vi "Car Wash.vi"() -> ()   [LabVIEW 2016, in "Car Wash.lvlib"]
uses:
  Car Wash.lvlib
  Controls/Car Wash Indicators.ctl
  Controls/Wash Options.ctl
  Controls/Queue Operations.ctl
  Controls/Data Cluster.ctl
  Controls/Timer Details.ctl
  Controls/Step Details.ctl
panel:
  out "Error Out":errorcluster
  in  "Start":bool
  out "Elapsed Time":dbl format="%0.2f"
  in  "stop":bool
  out "Wash Entry":bool
  in  "Wash Options":T1
  in  "Car Position":u8(slide) max=3 scale=0.0..4.0
  out "Car Wash Indicators":T2
  # "Entry Console"
  # "Car Wash Display"
  # "Car Position Simulation"
  # "Pre-Soak\nH-P Wash\nL-P Wax\nSpot Free Rinse"
  # "Underbody Wash\nBug Remover"
  # "Tire Shine\nAir Dry"
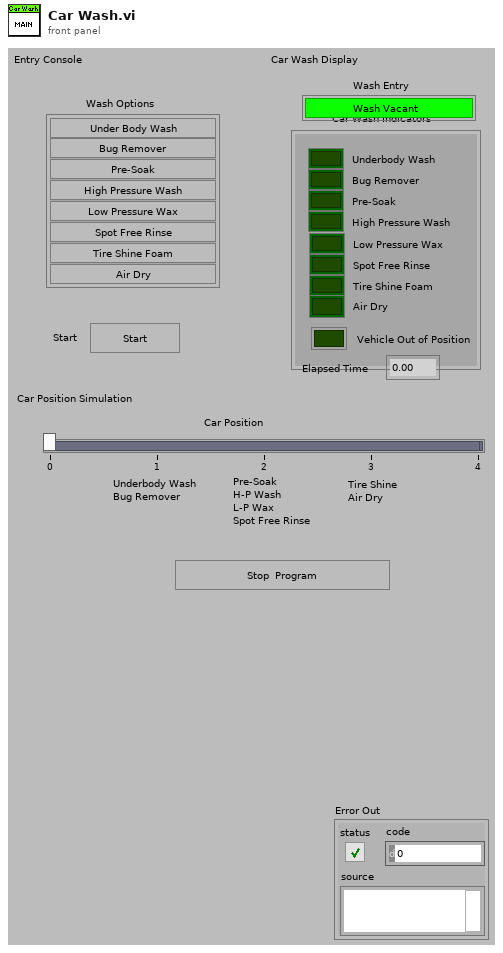
[diagram p1: front panel]
types:
  T1 = typedef "Car Wash.lvlib/Wash Options.ctl" = cluster{"Underbody Wash":bool, "Bug Remover":bool, "Pre-Soak":bool, "High Pressure Wash":bool, "Low Pressure Wax":bool, "Spot Free Rinse":bool, "Tire Shine Foam":bool, "Air Dry":bool}
  T2 = typedef "Car Wash.lvlib/Car Wash Indicators.ctl" = cluster{"Underbody Wash":bool, "Bug Remover":bool, "Pre-Soak":bool, "High Pressure Wash":bool, "Low Pressure Wax":bool, "Spot Free Rinse":bool, "Tire Shine Foam":bool, "Air Dry":bool, "Vehicle Out of Position":bool}
  T3 = typedef "Car Wash.lvlib/Data Cluster.ctl" = cluster{"Timer Details":T4, "Car Wash Indicators":T2, "Wash Options":T1, "Car Position Slider":u8, "Wash Entry":bool, "Enable Controls Ref":refnum<vi>[], "Disable Controls Ref":refnum<vi>[], "Steps Complete?":bool, "Selected Steps":T5[], "Current Step":T5, "Step Index (in selected)":i32, "Lookup":T5[]}
  T4 = typedef "Car Wash.lvlib/Timer Details.ctl" = cluster{"Paused?":bool, "Started?":bool, "Previous Time":timestamp, "Elapsed Time":dbl, "Set Time":dbl}
  T5 = typedef "Car Wash.lvlib/Step Details.ctl" = cluster{"Step":string, "Station":u8, "Time":dbl}
  T6 = typedef "Car Wash.lvlib/Queue Operations.ctl" = enum16{"Create", "Enqueue", "Enstack", "Dequeue", "Flush", "Release"}
  T7 = enum8{"Enabled", "Disabled", "Disabled and Grayed Out"}
  T8 = cluster{"Car Wash Indicators[0]":bool, "Car Wash Indicators[1]":bool, "Car Wash Indicators[2]":bool, "Car Wash Indicators[3]":bool, "Car Wash Indicators[4]":bool, "Car Wash Indicators[5]":bool, "Car Wash Indicators[6]":bool, "Car Wash Indicators[7]":bool, "Car Wash Indicators[8]":bool}
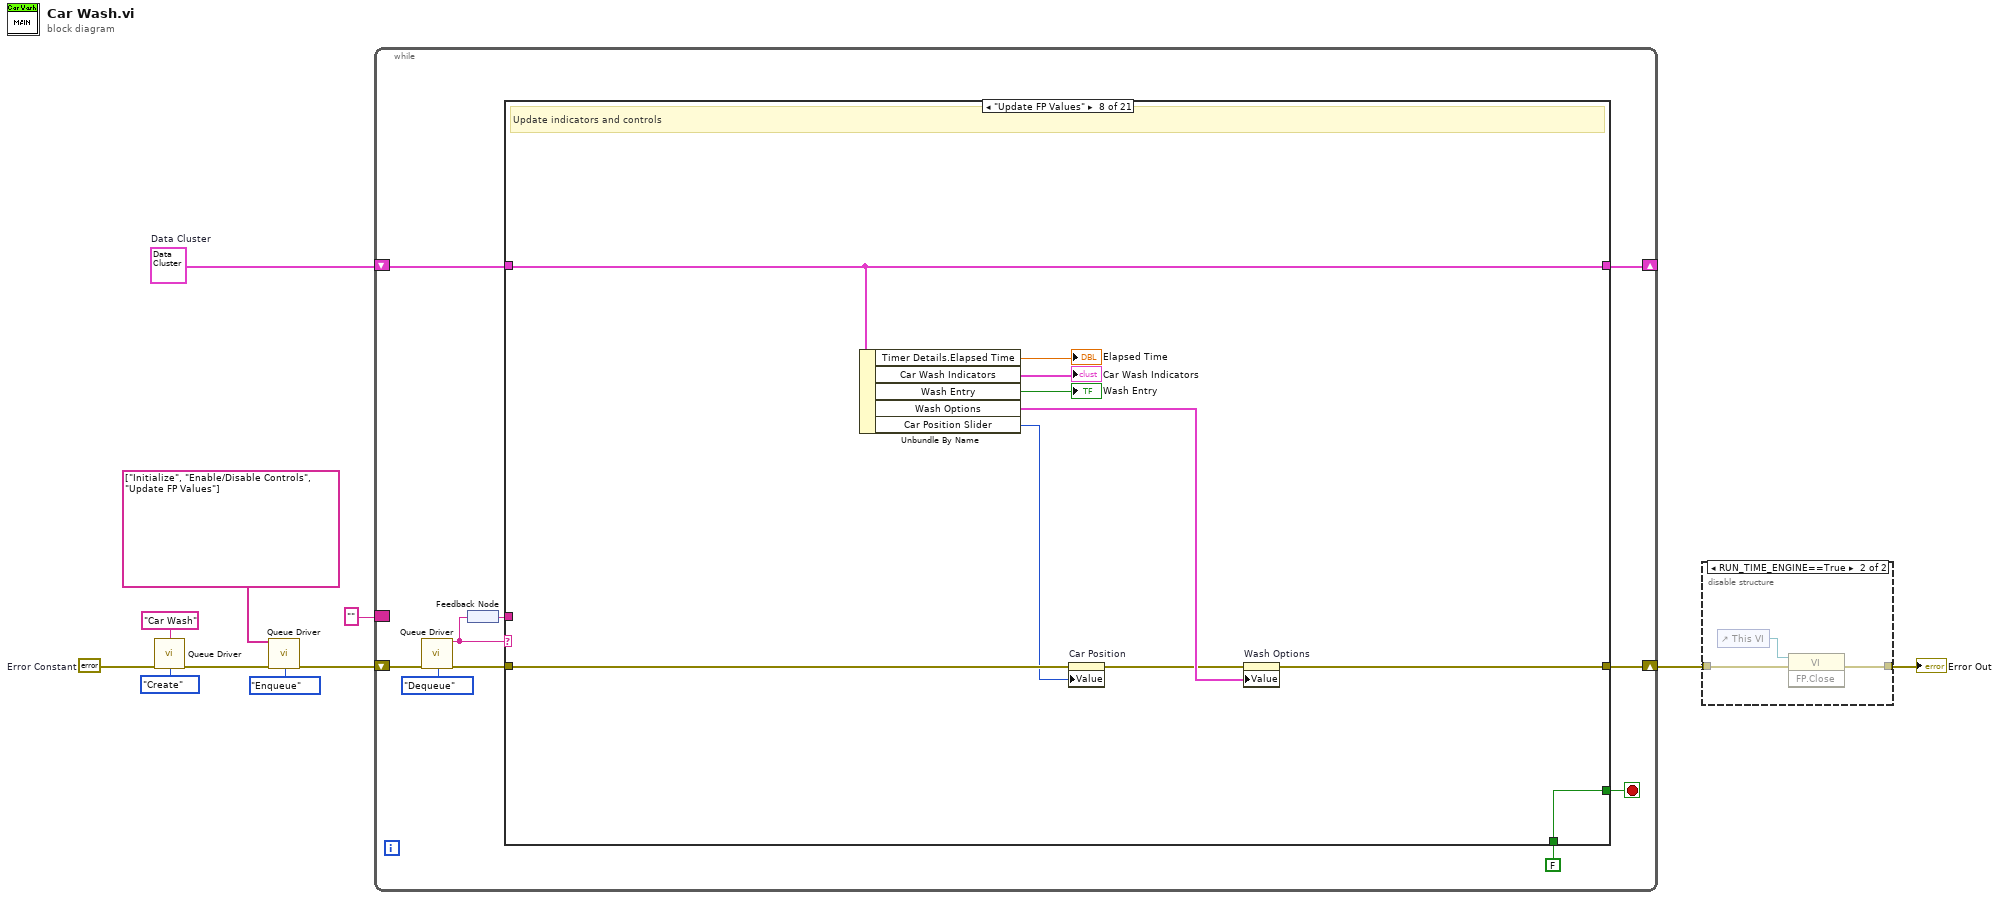
[diagram p0: block diagram]
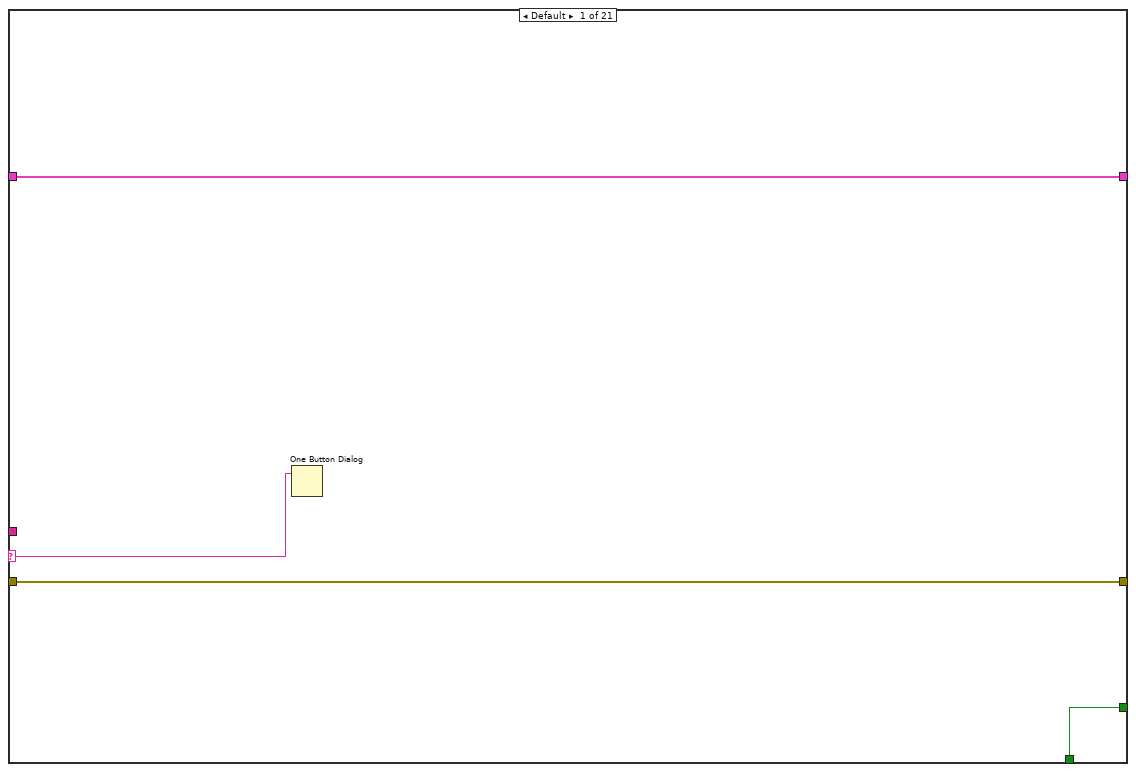
[diagram p2: hidden frame]
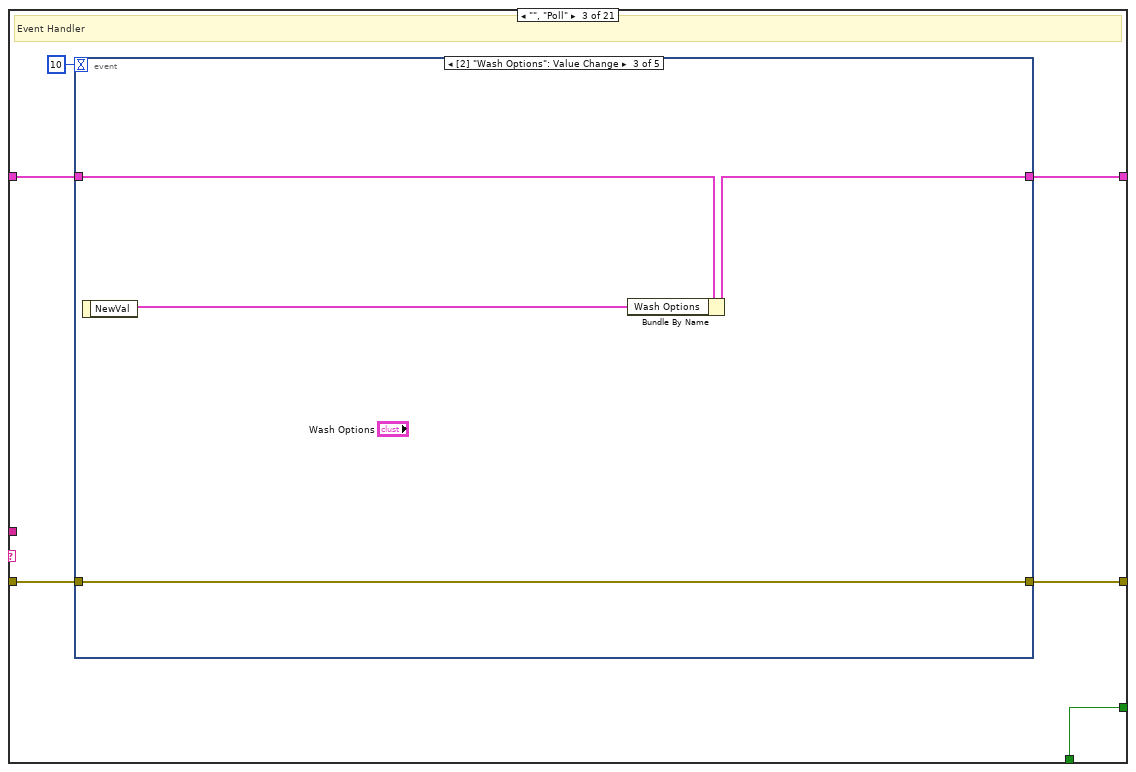
[diagram p4: hidden frame]
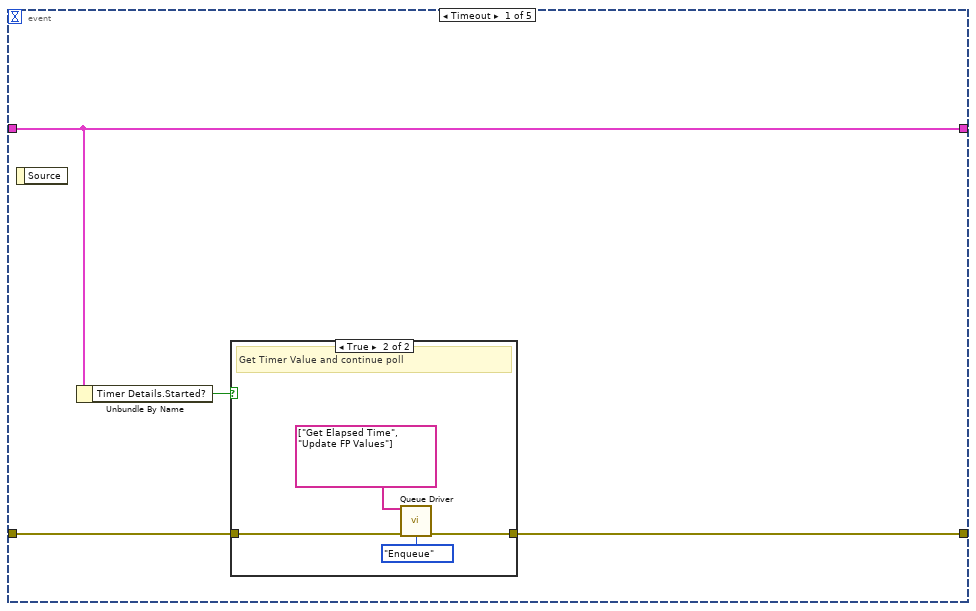
[diagram p5: hidden frame]
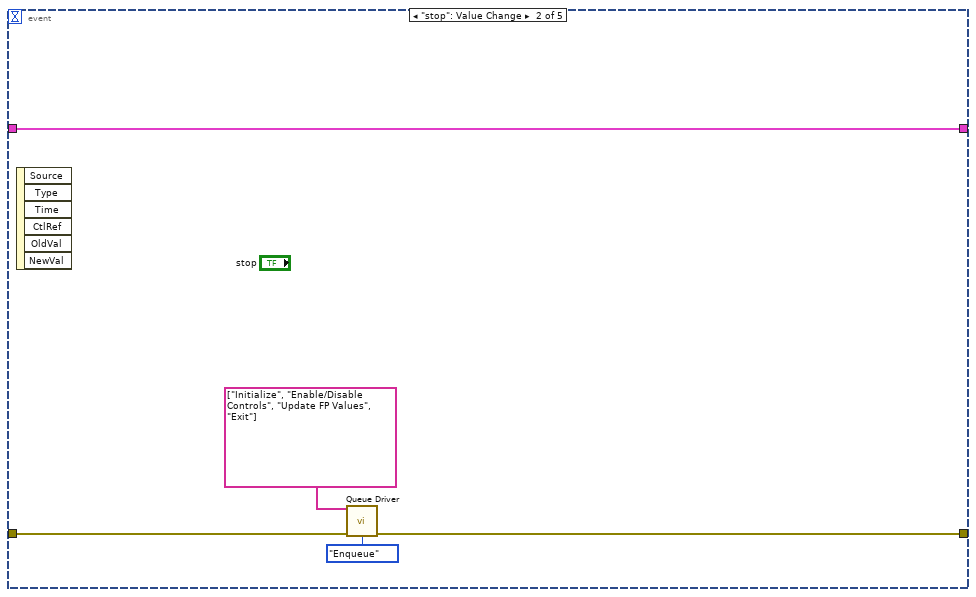
[diagram p7: hidden frame]
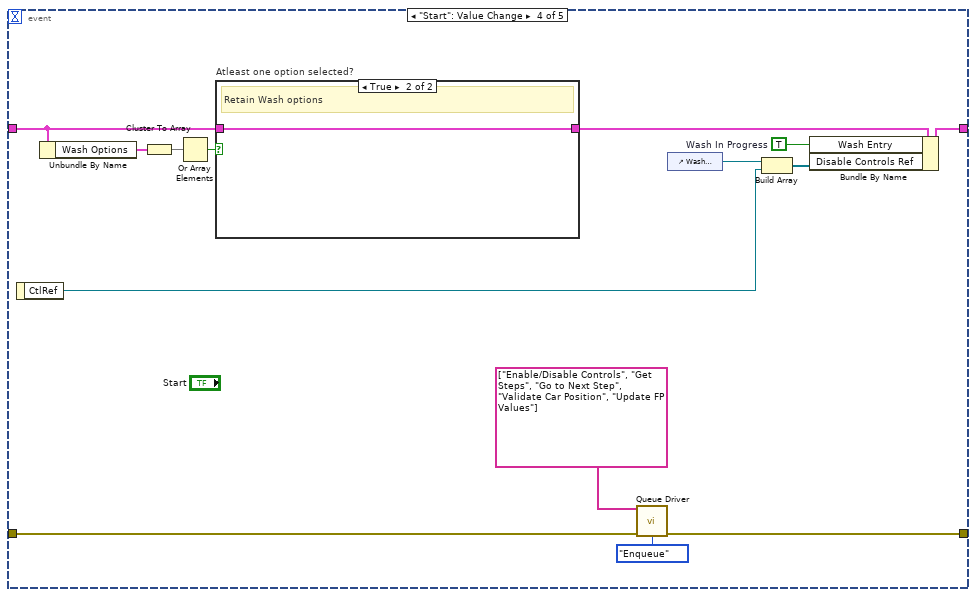
[diagram p8: hidden frame]
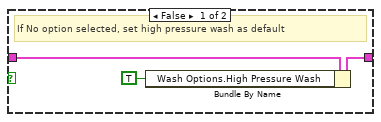
[diagram p9: hidden frame]
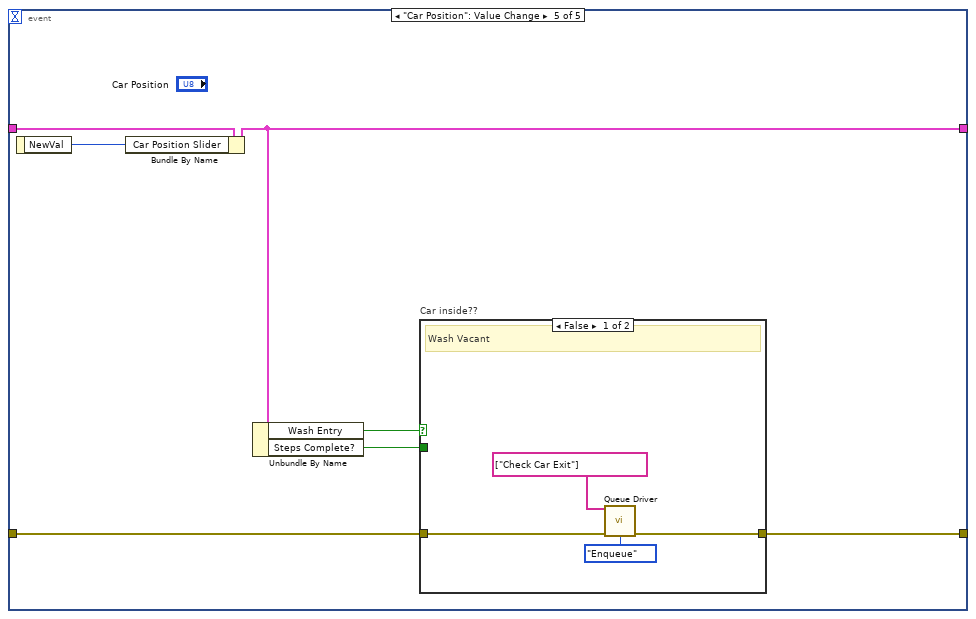
[diagram p10: hidden frame]
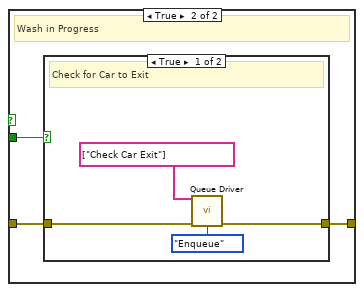
[diagram p11: hidden frame]
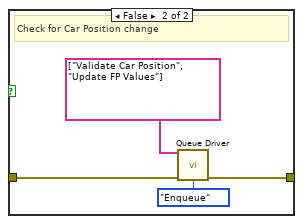
[diagram p12: hidden frame]
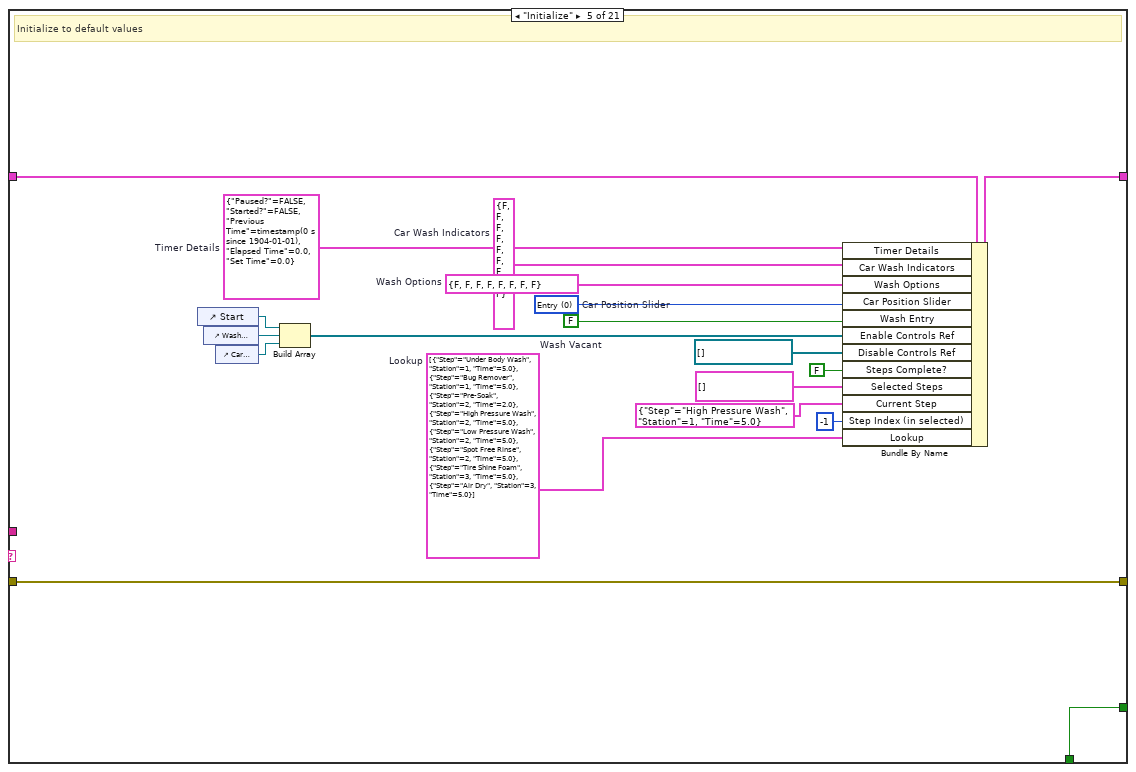
[diagram p14: hidden frame]
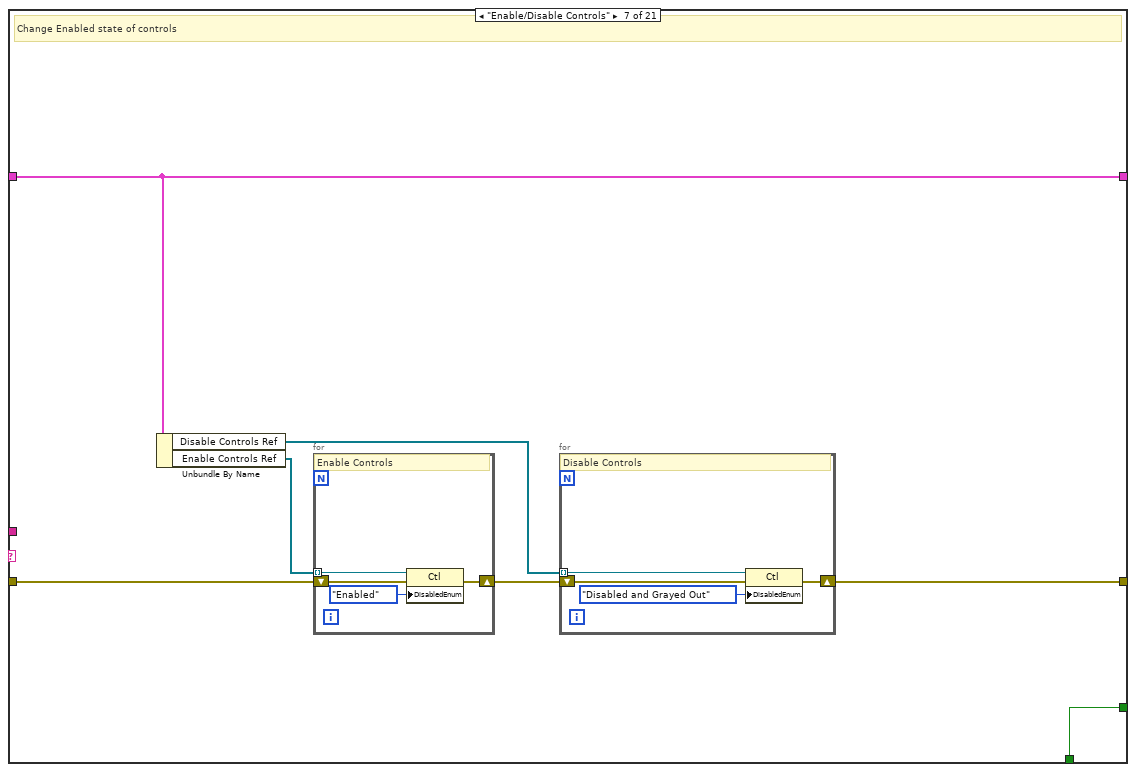
[diagram p16: hidden frame]
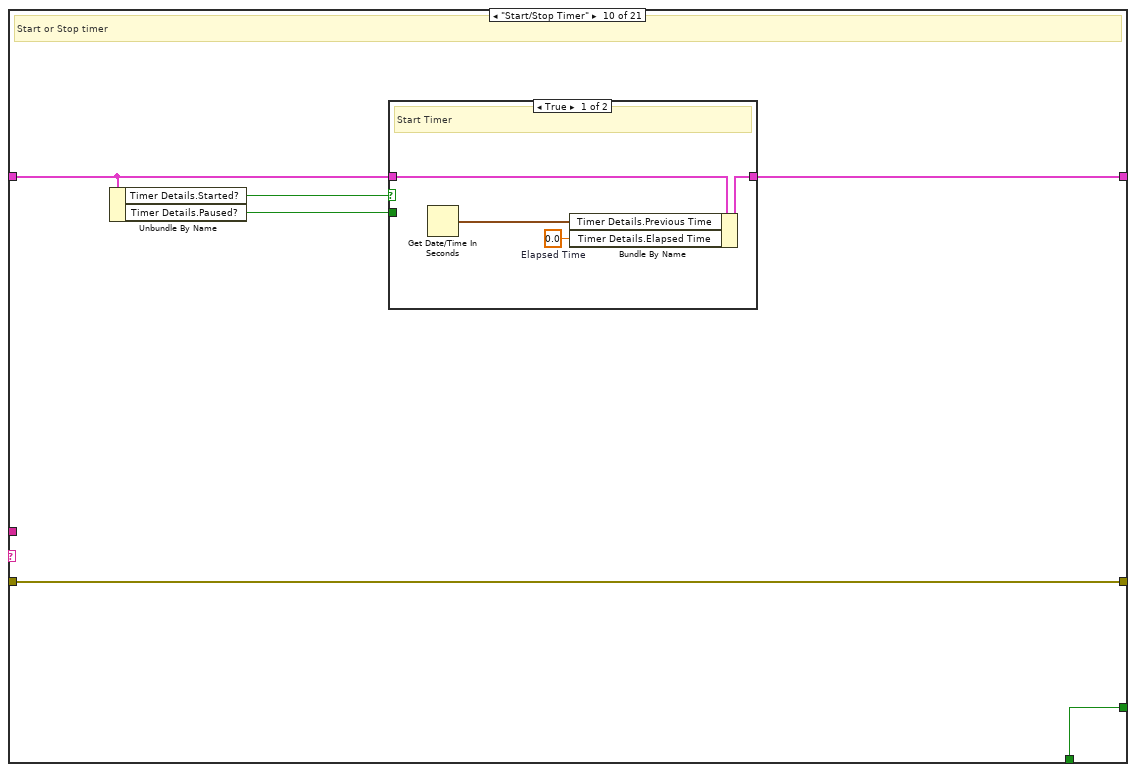
[diagram p18: hidden frame]
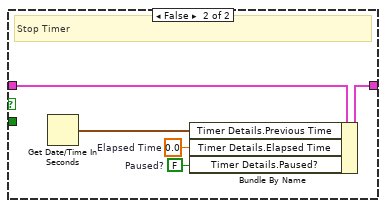
[diagram p19: hidden frame]
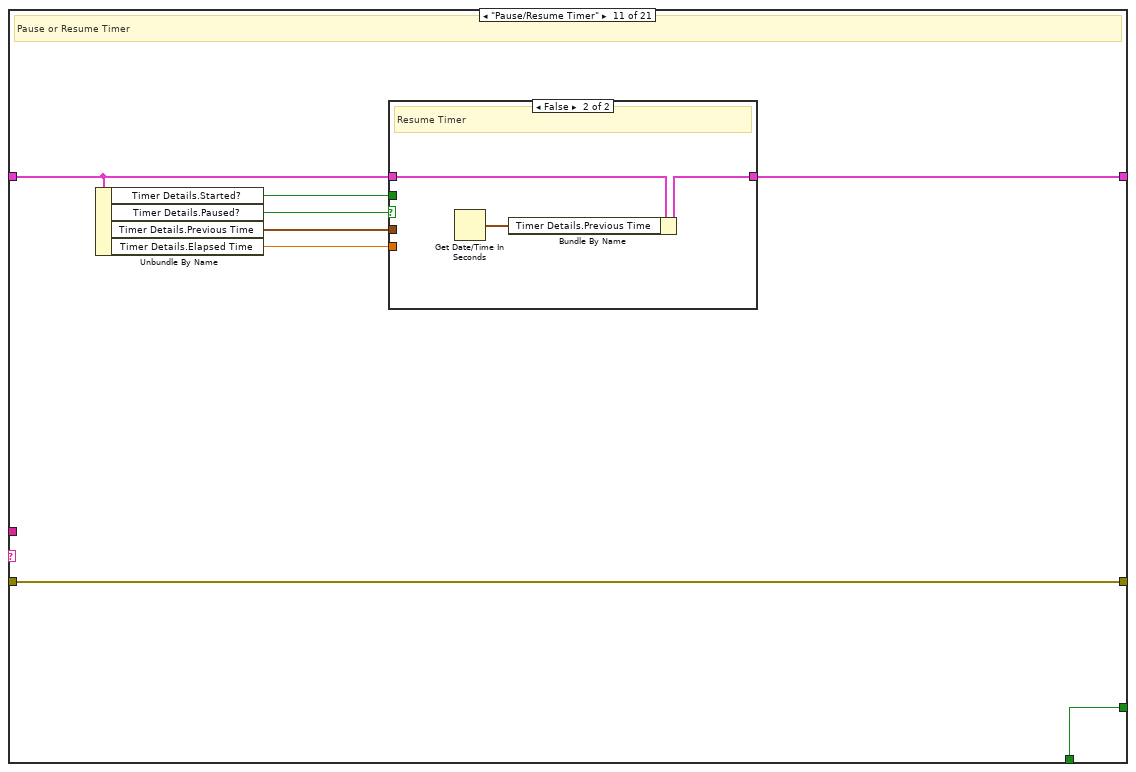
[diagram p20: hidden frame]
diagram:
  w3 = T3 {"Timer Details"={"Paused?"=FALSE, "Started?"=FALSE, "Previous Time"=timestamp(0 s since 1904-01-01), "Elapsed Time"=0.0, "Set Time"=0.0}, "Car Wash Indicators"={"Underbody Wash"=FALSE, "Bug Remover"=FALSE, "Pre-Soak"=FALSE, "High Pressure Wash"=FALSE, "Low Pressure Wax"=FALSE, "Spot Free Rinse"=FALSE, "Tire Shine Foam"=FALSE, "Air Dry"=FALSE, "Vehicle Out of Position"=FALSE}, "Wash Options"={"Underbody Wash"=FALSE, "Bug Remover"=FALSE, "Pre-Soak"=FALSE, "High Pressure Wash"=FALSE, "Low Pressure Wax"=FALSE, "Spot Free Rinse"=FALSE, "Tire Shine Foam"=FALSE, "Air Dry"=FALSE}, "Car Position Slider"=0, "Wash Entry"=FALSE, "Enable Controls Ref"=[], "Disable Controls Ref"=[], "Steps Complete?"=FALSE, "Selected Steps"=[], "Current Step"={"Step"="High Pressure Wash", "Station"=0, "Time"=0.0}, "Step Index (in selected)"=0, "Lookup"=[{"Step"="High Pressure Wash", "Station"=0, "Time"=0.0}, {"Step"="High Pressure Wash", "Station"=0, "Time"=0.0}, {"Step"="High Pressure Wash", "Station"=0, "Time"=0.0}, {"Step"="High Pressure Wash", "Station"=0, "Time"=0.0}, {"Step"="High Pressure Wash", "Station"=0, "Time"=0.0}, {"Step"="High Pressure Wash", "Station"=0, "Time"=0.0}, {"Step"="High Pressure Wash", "Station"=0, "Time"=0.0}, {"Step"="High Pressure Wash", "Station"=0, "Time"=0.0}]}  # Data Cluster
  w10 = errorcluster {"status"=FALSE, "code"=0, "source"=""}  # Error Constant
  n1 = call "Queue Driver.vi"("Queue Name"="Car Wash", "Error In"=w10, "Operation"=Queue_Operations."Create") -> ("Error Out"=w9:errorcluster)  [unwired: 11 in, 1 out]
  n2 = call "Queue Driver.vi"("Cases"=string[] ["Initialize", "Enable/Disable Controls", "Update FP Values"], "Error In"=w9, "Operation"=Queue_Operations."Enqueue") -> ("Error Out"=w8:errorcluster)  [unwired: 11 in, 1 out]
  n3 = while {
    shift-right: [w18] -> w2
    shift-left: w8 -> [w17]
    border: "" ("Dequeued Case") -> [_]
    shift-right: [w13] -> _
    shift-left: w3 -> [w14]
    stop <- w21 stop-if-true
    n4 = call "Queue Driver.vi"("Error In"=w17, "Operation"=Queue_Operations."Dequeue") -> ("Dequeued Case"=w16:string, "Error Out"=w19:errorcluster)  [unwired: 12 in]
    n5 = feedback #1() -> (w15:string)
    n6 = feedback-in #1(w16) -> ()
    n7 = case shown="\"Update FP Values\"" w16 {
      selector: w16 -> [w22 _ _ _ _ _ _ _ _ _ _ _ _ _ _ _ _ _ _ _ _]
      tunnel: FALSE -> [w25 w28 w34 w95 w114 w117 w124 w142 w145 w151 w168 w188 w203 w212 w226 w273 w301 w309 w323 w333 _]
      tunnel: [w25 w28 w34 w95 w114 w117 w124 w142 w145 w151 w168 w188 w203 w212 w226 w273 w301 w309 w323 w333 TRUE] -> w21
      tunnel: w19 -> [w24 w27 w33 w94 w113 w116 w121 w141 w144 w150 w167 w179 w202 w211 w220 w270 w298 w308 w322 w332 w340]
      tunnel: [w24 w27 w32 w94 w113 w116 w119 w136 w144 w150 w167 w178 w202 w211 w219 w269 w297 w308 w321 w332 w338] -> w18
      tunnel: w15 -> [_ _ _ _ _ _ _ _ _ _ _ _ _ _ _ _ _ _ w310 _ _]
      tunnel: w14 -> [w23 w26 w31 w93 w112 w115 w123 w140 w143 w147 w166 w185 w201 w207 w222 w272 w300 w307 w311 w331 w334]
      tunnel: [w23 w26 w30 w93 w111 w115 w123 w140 w143 w146 w165 w184 w201 w206 w221 w271 w300 w307 w311 w331 w334] -> w13
      frame Default {
        n8 = One Button Dialog(message=w22) -> ()  [unwired: 1 in, 1 out]
      }
      frame "----Poll----" {
      }
      frame "", "Poll" {
        # "Event Handler"
        n9 = event shown="[2] \"Wash Options\": Value Change" {
          selector: _ -> [_ _ _ _ _]
          dyn-events: _ -> [_ _ _ _ _]
          timeout: 10 -> [_ _ _ _ _]
          tunnel: w33 -> [w38 w47 w49 w60 w75]
          tunnel: [w37 w46 w49 w59 w74] -> w32
          tunnel: w31 -> [w36 w44 w52 w65 w77]
          tunnel: [w36 w44 w51 w57 w73] -> w30
          event Timeout {
            n10 = event-data() -> ()  [unwired: 1 in, 1 out]
            n11 = Unbundle By Name(w36) -> ("Timer Details.Started?"=w35:bool)
            n12 = case shown="True" w35 {
              tunnel: w38 -> [w39 w43]
              tunnel: [w39 w42] -> w37
              frame False {
                # "Timer Not Running, so keep polling"
              }
              frame True {
                # "Get Timer Value and continue poll"
                n13 = call "Queue Driver.vi"("Cases"=string[] ["Get Elapsed Time", "Update FP Values"], "Error In"=w43, "Operation"=Queue_Operations."Enqueue") -> ("Error Out"=w42:errorcluster)  [unwired: 11 in, 1 out]
              }
            }
          }
          event "stop": Value Change {
            n14 = event-data() -> ()  [unwired: 1 in, 6 out]
            n15 = call "Queue Driver.vi"("Cases"=string[] ["Initialize", "Enable/Disable Controls", "Update FP Values", "Exit"], "Error In"=w47, "Operation"=Queue_Operations."Enqueue") -> ("Error Out"=w46:errorcluster)  [unwired: 11 in, 1 out]
          }
          event Value Change {
            n16 = event-data() -> ("NewVal"=w50:T1)  [unwired: 1 in]
            n17 = Bundle By Name(cluster=w52, "Wash Options"=w50) -> (w51:T3)
          }
          event "Start": Value Change {
            w56 = TRUE  # Wash In Progress
            n18 = event-data() -> ("CtlRef"=w53:refnum<vi>)  [unwired: 1 in]
            n19 = Unbundle By Name(w65) -> ("Wash Options"=w63:T1)
            n20 = Cluster To Array(cluster=w63) -> (array=w64:bool[])
            n21 = Or Array Elements(Boolean array=w64) -> (logical OR=w62:bool)
            n22 = case "Atleast one option selected?" shown="True" w62 {
              tunnel: [w69 w70] -> w66
              tunnel: w65 -> [w68 w70]
              frame False {
                # "If No option selected, set high pressure wash as default"
                n23 = Bundle By Name(cluster=w68, "Wash Options.High Pressure Wash"=TRUE) -> (w69:T3)
              }
              frame True {
                # "Retain Wash options"
              }
            }
            n24 = call "Queue Driver.vi"("Cases"=string[] ["Enable/Disable Controls", "Get Steps", "Go to Next Step", "Validate Car Position", "Update FP Values"], "Error In"=w60, "Operation"=Queue_Operations."Enqueue") -> ("Error Out"=w59:errorcluster)  [unwired: 11 in, 1 out]
            n25 = control-ref of="Wash Options"() -> (w55:refnum<vi>)
            n26 = Build Array(w55, w53) -> (w54:refnum<vi>[])
            n27 = Bundle By Name(cluster=w66, "Wash Entry"=w56, "Disable Controls Ref"=w54) -> (w57:T3)
          }
          event "Car Position": Value Change {
            n28 = event-data() -> ("NewVal"=w76:u8)  [unwired: 1 in]
            n29 = Bundle By Name(cluster=w77, "Car Position Slider"=w76) -> (w73:T3)
            n30 = Unbundle By Name(w73) -> ("Wash Entry"=w71:bool, "Steps Complete?"=w72:bool)
            n31 = case "Car inside??" shown="False" w71 {
              tunnel: w75 -> [w81 w84]
              tunnel: [w80 w83] -> w74
              tunnel: w72 -> [_ w82]
              frame False {
                # "Wash Vacant"
                n32 = call "Queue Driver.vi"("Cases"=string[] ["Check Car Exit"], "Error In"=w81, "Operation"=Queue_Operations."Enqueue") -> ("Error Out"=w80:errorcluster)  [unwired: 11 in, 1 out]
              }
              frame True {
                # "Wash in Progress"
                n33 = case shown="True" w82 {
                  tunnel: w84 -> [w86 w90]
                  tunnel: [w85 w89] -> w83
                  frame True {
                    # "Check for Car to Exit"
                    n34 = call "Queue Driver.vi"("Cases"=string[] ["Check Car Exit"], "Error In"=w86, "Operation"=Queue_Operations."Enqueue") -> ("Error Out"=w85:errorcluster)  [unwired: 11 in, 1 out]
                  }
                  frame False {
                    # "Check for Car Position change"
                    n35 = call "Queue Driver.vi"("Cases"=string[] ["Validate Car Position", "Update FP Values"], "Error In"=w90, "Operation"=Queue_Operations."Enqueue") -> ("Error Out"=w89:errorcluster)  [unwired: 11 in, 1 out]
                  }
                }
              }
            }
          }
        }
      }
      frame "----Initialize----" {
      }
      frame "Initialize" {
        w96 = T5[] [{"Step"="Under Body Wash", "Station"=1, "Time"=5.0}, {"Step"="Bug Remover", "Station"=1, "Time"=5.0}, {"Step"="Pre-Soak", "Station"=2, "Time"=2.0}, {"Step"="High Pressure Wash", "Station"=2, "Time"=5.0}, {"Step"="Low Pressure Wash", "Station"=2, "Time"=5.0}, {"Step"="Spot Free Rinse", "Station"=2, "Time"=5.0}, {"Step"="Tire Shine Foam", "Station"=3, "Time"=5.0}, {"Step"="Air Dry", "Station"=3, "Time"=5.0}]  # Lookup
        w106 = FALSE  # Wash Vacant
        w107 = u8 0 items=["Entry", "Station 1", "Station 2", "Station 3", "Exit"]  # Car Position Slider
        w108 = T1 {"Underbody Wash"=FALSE, "Bug Remover"=FALSE, "Pre-Soak"=FALSE, "High Pressure Wash"=FALSE, "Low Pressure Wax"=FALSE, "Spot Free Rinse"=FALSE, "Tire Shine Foam"=FALSE, "Air Dry"=FALSE}  # Wash Options
        w109 = T2 {"Underbody Wash"=FALSE, "Bug Remover"=FALSE, "Pre-Soak"=FALSE, "High Pressure Wash"=FALSE, "Low Pressure Wax"=FALSE, "Spot Free Rinse"=FALSE, "Tire Shine Foam"=FALSE, "Air Dry"=FALSE, "Vehicle Out of Position"=FALSE}  # Car Wash Indicators
        w110 = T4 {"Paused?"=FALSE, "Started?"=FALSE, "Previous Time"=timestamp(0 s since 1904-01-01), "Elapsed Time"=0.0, "Set Time"=0.0}  # Timer Details
        # "Initialize to default values"
        n36 = control-ref of="Start"() -> (w103:refnum<vi>)
        n37 = control-ref of="Wash Options"() -> (w105:refnum<vi>)
        n38 = control-ref of="Car Position"() -> (w104:refnum<vi>)
        n39 = Build Array(w103, w105, w104) -> (w102:refnum<vi>[])
        n40 = Bundle By Name(cluster=w112, "Timer Details"=w110, "Car Wash Indicators"=w109, "Wash Options"=w108, "Car Position Slider"=w107, "Wash Entry"=w106, "Enable Controls Ref"=w102, "Disable Controls Ref"=refnum<vi>[] [], "Steps Complete?"=FALSE, "Selected Steps"=T5[] [], "Current Step"=T5 {"Step"="High Pressure Wash", "Station"=1, "Time"=5.0}, "Step Index (in selected)"=-1, "Lookup"=w96) -> (w111:T3)
      }
      frame "----FP Related----" {
      }
      frame "Enable/Disable Controls" {
        # "Change Enabled state of controls"
        n41 = Unbundle By Name(w123) -> ("Disable Controls Ref"=w118:refnum<vi>[], "Enable Controls Ref"=w122:refnum<vi>[])
        n42 = for {
          tunnel: w122 -> [w132] mode=indexing
          shift-right: [w129] -> w120
          shift-left: w121 -> [w131]
          # "Enable Controls"
          n43 = property class="Ctl"(reference=w132, error in=w131, "DisabledEnum"=T7."Enabled" ("Disabled")) -> (error out=w129:errorcluster)  [unwired: 1 out]
        }
        n44 = for {
          tunnel: w118 -> [w128] mode=indexing
          shift-right: [w125] -> w119
          shift-left: w120 -> [w127]
          # "Disable Controls"
          n45 = property class="Ctl"(reference=w128, error in=w127, "DisabledEnum"=T7."Disabled and Grayed Out" ("Disabled")) -> (error out=w125:errorcluster)  [unwired: 1 out]
        }
      }
      frame "Update FP Values" {
        # "Update indicators and controls"
        n46 = Unbundle By Name(w140) -> ("Timer Details.Elapsed Time"=→"Elapsed Time":dbl, "Car Wash Indicators"=→"Car Wash Indicators":T2, "Wash Entry"=→"Wash Entry":bool, "Wash Options"=w135:T1, "Car Position Slider"=w133:u8)
        n47 = property on="Car Position" class="Slide (strict)"(error in=w141, "Value"=w133) -> (error out=w134:errorcluster)  [unwired: 1 in, 1 out]
        n48 = property on="Wash Options" class="Clust (strict)"(error in=w134, "Value"=w135) -> (error out=w136:errorcluster)  [unwired: 1 in, 1 out]
      }
      frame "----Timer----" {
      }
      frame "Start/Stop Timer" {
        # "Start or Stop timer"
        n49 = Unbundle By Name(w147) -> ("Timer Details.Started?"=w149:bool, "Timer Details.Paused?"=w148:bool)
        n50 = case shown="True" w149 {
          tunnel: w148 -> [_ _]
          tunnel: w147 -> [w155 w160]
          tunnel: [w154 w159] -> w146
          frame True {
            w152 = 0.0  # Elapsed Time
            # "Start Timer"
            n51 = Get Date/Time In Seconds() -> (seconds since 1Jan1904=w153:timestamp)
            n52 = Bundle By Name(cluster=w155, "Timer Details.Previous Time"=w153, "Timer Details.Elapsed Time"=w152) -> (w154:T3)
          }
          frame False {
            w156 = FALSE  # Paused?
            w157 = 0.0  # Elapsed Time
            # "Stop Timer"
            n53 = Get Date/Time In Seconds() -> (seconds since 1Jan1904=w158:timestamp)
            n54 = Bundle By Name(cluster=w160, "Timer Details.Previous Time"=w158, "Timer Details.Elapsed Time"=w157, "Timer Details.Paused?"=w156) -> (w159:T3)
          }
        }
      }
      frame "Pause/Resume Timer" {
        # "Pause or Resume Timer"
        n55 = Unbundle By Name(w166) -> ("Timer Details.Started?"=w162:bool, "Timer Details.Paused?"=w161:bool, "Timer Details.Previous Time"=w164:timestamp, "Timer Details.Elapsed Time"=w163:dbl)
        n56 = case shown="False" w161 {
          tunnel: w166 -> [w172 w175]
          tunnel: [w171 w174] -> w165
          tunnel: w164 -> [_ _]
          tunnel: w163 -> [w169 _]
          tunnel: w162 -> [_ _]
          frame True {
            # "Pause Timer"
            n57 = Get Date/Time In Seconds() -> (seconds since 1Jan1904=w170:timestamp)
            n58 = Bundle By Name(cluster=w172, "Timer Details.Previous Time"=w170, "Timer Details.Elapsed Time"=w169) -> (w171:T3)
          }
          frame False {
            # "Resume Timer"
            n59 = Get Date/Time In Seconds() -> (seconds since 1Jan1904=w173:timestamp)
            n60 = Bundle By Name(cluster=w175, "Timer Details.Previous Time"=w173) -> (w174:T3)
          }
        }
      }
      frame "Get Elapsed Time" {
        # "Elapsed Time (new) = Current time - Previous time + Elapsed Time(old)"
        # "Get the Elapsed Time"
        n61 = Unbundle By Name(w185) -> ("Timer Details.Paused?"=w176:bool, "Timer Details.Previous Time"=w187:timestamp, "Timer Details.Elapsed Time"=w186:dbl, "Timer Details.Set Time"=w181:dbl)
        n62 = case shown="False" w176 {
          tunnel: w187 -> [w193 w194]
          tunnel: w186 -> [w191 w195]
          tunnel: [w190 w194] -> w183
          tunnel: [w189 w195] -> w182
          frame False {
            # "Get the elapsed time"
            n63 = Get Date/Time In Seconds() -> (seconds since 1Jan1904=w190:timestamp)
            n64 = Subtract(x=w190, y=w193) -> (x-y=w192:dbl)
            n65 = Add(x=w192, y=w191) -> (x+y=w189:dbl)
          }
          frame True {
            # "Give same value if timer paused"
          }
        }
        n66 = Greater Or Equal?(x=w182, y=w181) -> (x >= y?=w180:bool)
        n67 = Not(x=w180) -> (.not. x?=w177:bool)
        n68 = case shown="False" w180 {
          tunnel: w179 -> [w196 w199]
          tunnel: [w196 w198] -> w178
          frame False {
            # "Continue current step"
          }
          frame True {
            # "Current Step Completed. Proceed to next step"
            n69 = call "Queue Driver.vi"("Cases"=string[] ["Start/Stop Timer", "Go to Next Step"], "Error In"=w199, "Operation"=Queue_Operations."Enqueue") -> ("Error Out"=w198:errorcluster)  [unwired: 11 in, 1 out]
          }
        }
        n70 = Bundle By Name(cluster=w185, "Timer Details.Previous Time"=w183, "Timer Details.Elapsed Time"=w182, "Timer Details.Started?"=w177) -> (w184:T3)
      }
      frame "----Functionality----" {
      }
      frame "Get Steps" {
        # "Get the list of selected steps"
        n71 = Unbundle By Name(w207) -> ("Lookup"=w209:T5[], "Wash Options"=w210:T1)
        n72 = Cluster To Array(cluster=w210) -> (array=w208:bool[])
        n73 = for "Get Selected Steps" {
          tunnel: w209 -> [w214] mode=indexing
          tunnel: w208 -> [w213] mode=indexing
          tunnel: [w214] -> w205 mode=indexing if=w213
        }
        n74 = Bundle By Name(cluster=w207, "Selected Steps"=w205, "Step Index (in selected)"=-1) -> (w206:T3)
      }
      frame "Validate Car Position" {
        # "Check for Out of Position"
        n75 = Unbundle By Name(w222) -> ("Car Position Slider"=w225:u8, "Current Step.Station"=w224:u8, "Car Wash Indicators"=w218:T2, "Lookup"=w217:T5[], "Current Step"=w216:T5)
        n76 = Equal?(x=w225, y=w224) -> (x = y?=w223:bool)
        n77 = Search 1D Array(1D array=w217, element=w216) -> (index of element=w215:i32)  [unwired: 1 in]
        n78 = case shown="False" w223 {
          tunnel: w222 -> [w241 w248]
          tunnel: [w240 w247] -> w221
          tunnel: w220 -> [w237 w256]
          tunnel: [w236 w255] -> w219
          tunnel: w218 -> [w235 w246]
          tunnel: w215 -> [w233 w245]
          frame True {
            w232 = 8  # Out of Position
            w227 = FALSE  # Resume
            # "increment on adding additional wash steps to the software"
            # "Resume the timer"
            # "change cluster size on adding additional wash steps to the software"
            # "Vehicle in required position"
            n79 = Cluster To Array(cluster=w235) -> (array=w234:bool[])
            n80 = in-place {
              # "update Step indicator= T and\nOut of position = F"
              n81 = in-place-array #2(w234, w233, w232) -> ()  [unwired: 2 out]
              n82 = in-place-array #2(TRUE ("element"), FALSE ("Timer Details.Paused?")) -> (w231:bool[])  [unwired: 2 out]
            }
            n83 = Array To Cluster(array=w231) -> (cluster=w230:T8)
            n84 = Type Cast(type=T2 {"Underbody Wash"=FALSE, "Bug Remover"=FALSE, "Pre-Soak"=FALSE, "High Pressure Wash"=FALSE, "Low Pressure Wax"=FALSE, "Spot Free Rinse"=FALSE, "Tire Shine Foam"=FALSE, "Air Dry"=FALSE, "Vehicle Out of Position"=FALSE} ("Car Wash Indicators"), x=w230) -> (*(type *) &x=w229:T2)
            n85 = Bundle By Name(cluster=w241, "Car Wash Indicators"=w229, "Timer Details.Paused?"=w227) -> (w240:T3)
            n86 = call "Queue Driver.vi"("Cases"=string[] ["Pause/Resume Timer", "Update FP Values"], "Error In"=w237, "Operation"=Queue_Operations."Enqueue") -> ("Error Out"=w236:errorcluster)  [unwired: 11 in, 1 out]
          }
          frame False {
            w253 = 8  # Out of Position
            w244 = TRUE  # Pause
            # "increment on adding additional wash steps to the software"
            # "Pause the timer"
            # "change cluster size on adding additional wash steps to the software"
            # "Vehicle not in required position"
            n87 = Cluster To Array(cluster=w246) -> (array=w254:bool[])
            n88 = in-place {
              # "update Step indicator= F and\nOut of position = T"
              n89 = in-place-array #3(w254, w245, w253) -> ()  [unwired: 2 out]
              n90 = in-place-array #3(FALSE ("element"), TRUE ("Timer Details.Paused?")) -> (w252:bool[])  [unwired: 2 out]
            }
            n91 = Array To Cluster(array=w252) -> (cluster=w251:T8)
            n92 = Type Cast(type=T2 {"Underbody Wash"=FALSE, "Bug Remover"=FALSE, "Pre-Soak"=FALSE, "High Pressure Wash"=FALSE, "Low Pressure Wax"=FALSE, "Spot Free Rinse"=FALSE, "Tire Shine Foam"=FALSE, "Air Dry"=FALSE, "Vehicle Out of Position"=FALSE} ("Car Wash Indicators"), x=w251) -> (*(type *) &x=w250:T2)
            n93 = call "Queue Driver.vi"("Cases"=string[] ["Pause/Resume Timer", "Update FP Values"], "Error In"=w256, "Operation"=Queue_Operations."Enqueue") -> ("Error Out"=w255:errorcluster)  [unwired: 11 in, 1 out]
            n94 = Bundle By Name(cluster=w248, "Car Wash Indicators"=w250, "Timer Details.Paused?"=w244) -> (w247:T3)
          }
        }
      }
      frame "Go to Next Step" {
        # "Start the next wash step"
        n95 = Unbundle By Name(w272) -> ("Lookup"=w262:T5[], "Current Step"=w261:T5, "Selected Steps"=w268:T5[], "Step Index (in selected)"=w266:i32)  [unwired: 2 out]
        n96 = Array Size(array=w268) -> (size(s)=w267:i32)
        n97 = Increment(x=w266) -> (x+1=w263:i32)
        n98 = Decrement(x=w267) -> (x-1=w265:i32)
        n99 = Greater Or Equal?(x=w265, y=w263) -> (x >= y?=w264:bool)
        n100 = case "Steps remaining?" shown="True" w264 {
          tunnel: w272 -> [w287 w296]
          tunnel: [w286 w295] -> w271
          tunnel: w270 -> [w285 w294]
          tunnel: [w284 w293] -> w269
          tunnel: w268 -> [w283 _]
          tunnel: w263 -> [w282 _]
          tunnel: w262 -> [w277 _]
          tunnel: w261 -> [w276 _]
          frame True {
            w278 = T2 {"Underbody Wash"=FALSE, "Bug Remover"=FALSE, "Pre-Soak"=FALSE, "High Pressure Wash"=FALSE, "Low Pressure Wax"=FALSE, "Spot Free Rinse"=FALSE, "Tire Shine Foam"=FALSE, "Air Dry"=FALSE, "Vehicle Out of Position"=FALSE}  # Default
            w279 = TRUE  # Start
            # "Start Next Step"
            n101 = Search 1D Array(1D array=w277, element=w276) -> ()  [unwired: 1 in, 1 out]
            n102 = Index Array(array=w283, index=w282) -> (element=w275:T5)
            n103 = Unbundle By Name(w275) -> ("Time"=w274:dbl)
            n104 = Bundle By Name(cluster=w287, "Car Wash Indicators"=w278, "Current Step"=w275, "Step Index (in selected)"=w282, "Timer Details.Started?"=w279, "Timer Details.Set Time"=w274) -> (w286:T3)
            n105 = call "Queue Driver.vi"("Cases"=string[] ["Start/Stop Timer", "Validate Car Position"], "Error In"=w285, "Operation"=Queue_Operations."Enqueue") -> ("Error Out"=w284:errorcluster)  [unwired: 11 in, 1 out]
          }
          frame False {
            w288 = TRUE  # Steps Completed
            w289 = T2 {"Underbody Wash"=FALSE, "Bug Remover"=FALSE, "Pre-Soak"=FALSE, "High Pressure Wash"=FALSE, "Low Pressure Wax"=FALSE, "Spot Free Rinse"=FALSE, "Tire Shine Foam"=FALSE, "Air Dry"=FALSE, "Vehicle Out of Position"=TRUE}  # Vehicle Out of Position
            # "Set Out of Position and Wait for Car Exit"
            n106 = call "Queue Driver.vi"("Cases"=string[] ["Update FP Values"], "Error In"=w294, "Operation"=Queue_Operations."Enqueue") -> ("Error Out"=w293:errorcluster)  [unwired: 11 in, 1 out]
            n107 = Bundle By Name(cluster=w296, "Car Wash Indicators"=w289, "Step Index (in selected)"=-1, "Steps Complete?"=w288) -> (w295:T3)
          }
        }
      }
      frame "Check Car Exit" {
        # "Check for exit of car and reinitialize"
        n108 = Unbundle By Name(w300) -> ("Car Position Slider"=w299:u8)
        n109 = case shown="Default" w299 {
          tunnel: w298 -> [w302 w303]
          tunnel: [w302 w304] -> w297
          frame Default {
          }
          frame 4 {
            # "Change the case number when adding additional positions to the software"
            # "Car Reached Exit. Reinitialize controls to default state"
            n110 = call "Queue Driver.vi"("Cases"=string[] ["Initialize", "Enable/Disable Controls", "Update FP Values"], "Error In"=w303, "Operation"=Queue_Operations."Enqueue") -> ("Error Out"=w304:errorcluster)  [unwired: 11 in, 1 out]
          }
        }
      }
      frame "----Error----" {
      }
      frame "Error" {
        # "Handle errors"
        n111 = Unbundle By Name(w322) -> ("code"=w317:i32, "source"=w316:string)
        n112 = call <vilib>:"Clear Errors.vi"("error in (no error)"=w322, "specific error code to clear (0: all)"=w317) -> ("error out"=w320:errorcluster)  [unwired: 4 in, 1 out]
        n113 = Format Into String(format string="Error occurred in state \"%s\"!!\nError Code: %d\nError Source: %s\n\nDo you wish to continue?", error in=w320, w310, w317, w316) -> (resulting string=w315:string, error out=w319:errorcluster)  [unwired: 1 in]
        n114 = Two Button Dialog(message=w315, 1:"Exit" ("F button name (\"Cancel\")"), 2:"Continue" ("T button name (\"OK\")")) -> (T button?=w312:bool)
        n115 = case shown="False" w312 {
          tunnel: w319 -> [w324 w327]
          tunnel: [w324 w325] -> w321
          frame True {
            # "Continue"
          }
          frame False {
            # "Exit"
            n116 = call "Queue Driver.vi"("Error In"=w327, "Operation"=Queue_Operations."Flush") -> ("Error Out"=w326:errorcluster)  [unwired: 12 in, 1 out]
            n117 = call "Queue Driver.vi"("Cases"=string[] ["Initialize", "Enable/Disable Controls", "Update FP Values", "Exit"], "Error In"=w326, "Operation"=Queue_Operations."Enqueue") -> ("Error Out"=w325:errorcluster)  [unwired: 11 in, 1 out]
          }
        }
      }
      frame "----Exit----" {
      }
      frame "Exit" {
        # "Exit the State Machine"
        n118 = call "Queue Driver.vi"("Error In"=w340, "Operation"=Queue_Operations."Flush") -> ("Error Out"=w339:errorcluster)  [unwired: 12 in, 1 out]
        n119 = call "Queue Driver.vi"("Error In"=w339, "Operation"=Queue_Operations."Release") -> ("Error Out"=w338:errorcluster)  [unwired: 12 in, 1 out]
      }
    }
  }
  n120 = disable-structure shown="RUN_TIME_ENGINE==True" {
    disable-tunnel: w2 -> [w341 w344]
    disable-tunnel: [w341 w343] -> w1
    frame condition #0 (active) {
    }
    frame condition #1 {
      n121 = control-ref of="This VI"() -> (w342:refnum<vi>)
      n122 = invoke class="VI" method="FP.Close"(reference=w342, error in=w344) -> (error out=w343:errorcluster)  [unwired: 1 in, 2 out]
    }
  }
  "Error Out" <- w1
